vi "Get lsl stream Info.vi"() -> ()   [LabVIEW 2016, in "Lab Streaming Layer.lvlib"]
uses:
  Lab Streaming Layer.lvlib
  Custom Controls/lsl_channel_format.ctl
  Custom Controls/lsl_xml_ptr.ctl
panel:
  out "source id":string
  out "nominal samplerate":dbl
  out "hostname":string
  out "xml_ptr":T1
  out "name":string
  out "created at":dbl
  out "channel bytes":i32
  out "channel count":i32
  out "xml":string
  out "version":i32
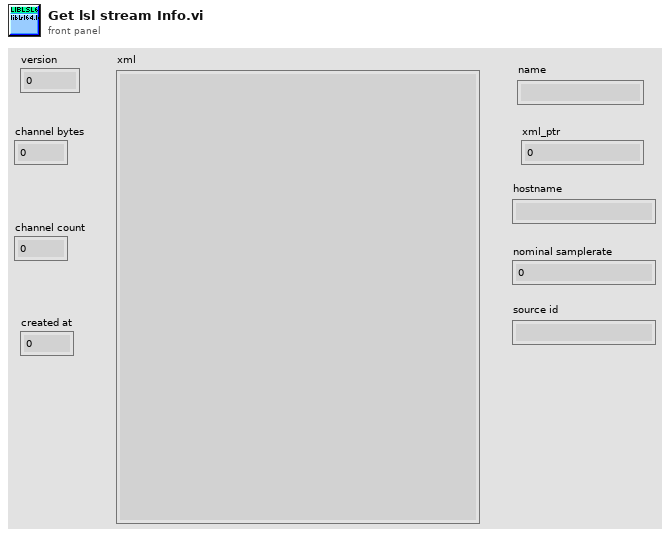
[diagram p1: front panel]
types:
  T1 = typedef "liblsl-LabVIEW.lvlib/lsl_xml_ptr.ctl" = u64
  T2 = typedef "liblsl-LabVIEW.lvlib/lsl_channel_format.ctl" = u32
  T3 = typedef "liblsl-LabVIEW.lvlib/lsl_streaminfo.ctl" = u64
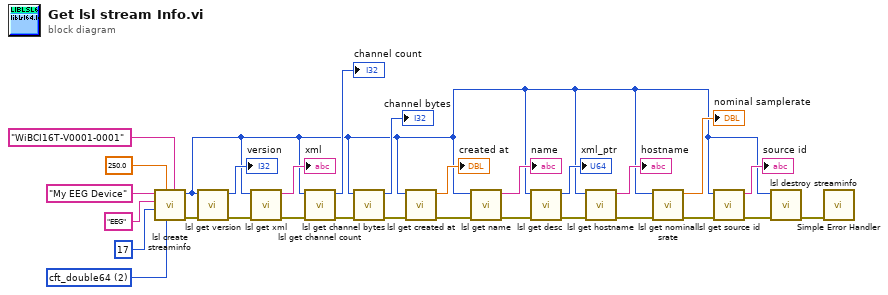
[diagram p0: block diagram]
diagram:
  w24 = T2 2 items=["cft_float32"=1, "cft_double64"=2, "cft_string"=3, "cft_int32"=4, "cft_int16"=5, "cft_int8"=6, "cft_int64"=7, "cft_undefined"=0] ("channel_format")
  n1 = call "lsl create streaminfo.vi"("source_id"="WiBCI16T-V0001-0001", "channel_format"=w24, "samplingrate"=250.0, "channel_count"=17, "type"="EEG", "name"="My EEG Device") -> ("error out"=w23:errorcluster, "streaminfo"=w3:T3)  [unwired: 4 in]
  n2 = call "lsl get version.vi"("error in (no error)"=w23, "streaminfo"=w3) -> ("error out"=w22:errorcluster, "version"=→"version":i32)  [unwired: 8 in]
  n3 = call "lsl get xml.vi"("error in (no error)"=w22, "streaminfo"=w3) -> ("error out"=w19:errorcluster, "xml"=→"xml":string)  [unwired: 8 in]
  n4 = call "lsl get channel count.vi"("error in (no error)"=w19, "streaminfo"=w3) -> ("error out"=w17:errorcluster, "channel count"=→"channel count":i32)  [unwired: 8 in]
  n5 = call "lsl get channel bytes.vi"("error in (no error)"=w17, "streaminfo"=w3) -> ("error out"=w15:errorcluster, "channel bytes"=→"channel bytes":i32)  [unwired: 8 in]
  n6 = call "lsl get created at.vi"("error in (no error)"=w15, "streaminfo"=w3) -> ("error out"=w13:errorcluster, "created at"=→"created at":dbl)  [unwired: 8 in]
  n7 = call "lsl get name.vi"("error in (no error)"=w13, "streaminfo"=w3) -> ("error out"=w11:errorcluster, "name"=→"name":string)  [unwired: 8 in]
  n8 = call "lsl get desc.vi"("error in (no error)"=w11, "streaminfo"=w3) -> ("error out"=w9:errorcluster, "xml_ptr"=→"xml_ptr":T1)  [unwired: 8 in]
  n9 = call "lsl get hostname.vi"("error in (no error)"=w9, "streaminfo"=w3) -> ("error out"=w7:errorcluster, "hostname"=→"hostname":string)  [unwired: 8 in]
  n10 = call "lsl get nominal srate.vi"("error in (no error)"=w7, "streaminfo"=w3) -> ("error out"=w5:errorcluster, "nominal samplerate"=→"nominal samplerate":dbl)  [unwired: 8 in]
  n11 = call "lsl get source id.vi"("error in (no error)"=w5, "streaminfo"=w3) -> ("error out"=w2:errorcluster, "source id"=→"source id":string)  [unwired: 8 in]
  n12 = call "lsl destroy streaminfo.vi"("error in (no error)"=w2, "streaminfo"=w3) -> ("error out"=w1:errorcluster)  [unwired: 9 in]
  n13 = call <vilib>:"Simple Error Handler.vi"("error in (no error)"=w1) -> ()  [unwired: 4 in, 5 out]
